vi "Writedata_spectra_normonly.vi"(0 "tdms file in":refnum<k34>, 1 "Aquisition number":i32, 2 "Norm Visible Intensity":cluster{dbl[], dbl[]}(graph)={array[2028 elements], array[2028 elements]}, 3 "tdms error in":errorcluster, 4 "Params":T1) -> (5 "tdms file out":refnum<k34>, 6 "tdms error out":errorcluster)   [LabVIEW 2018]
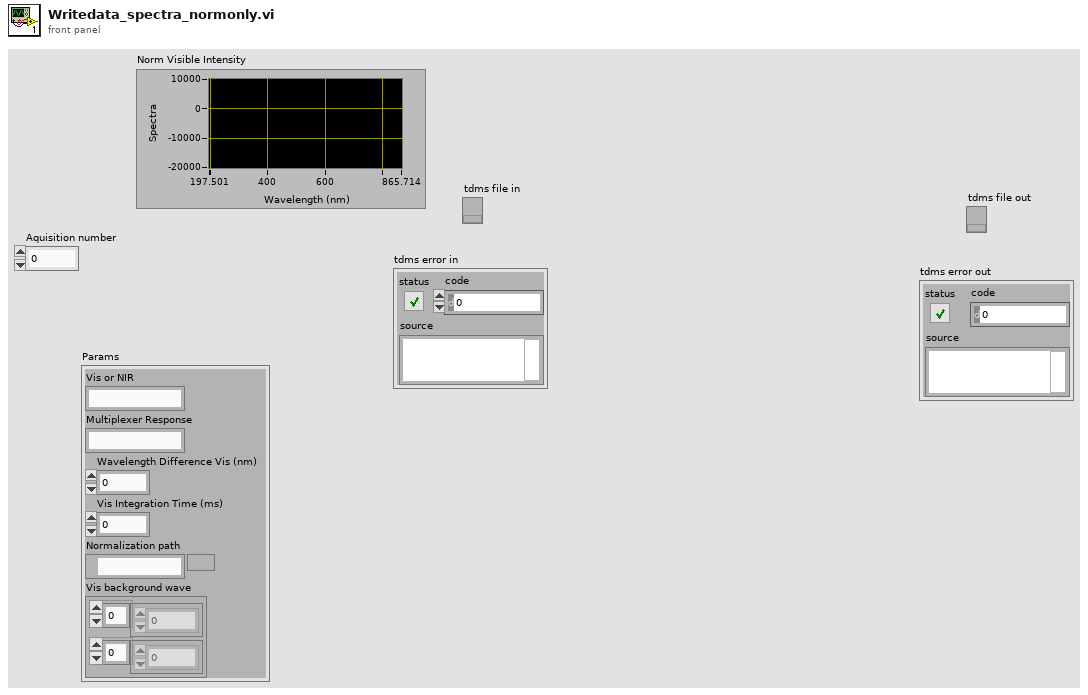
[diagram p1: front panel]
types:
  T1 = cluster{"Vis or NIR":string, "Multiplexer Response":string, "Wavelength Difference Vis (nm)":dbl, "Vis Integration Time (ms)":u32, "Normalization path":path, "Vis background wave":cluster{dbl[], dbl[]}}
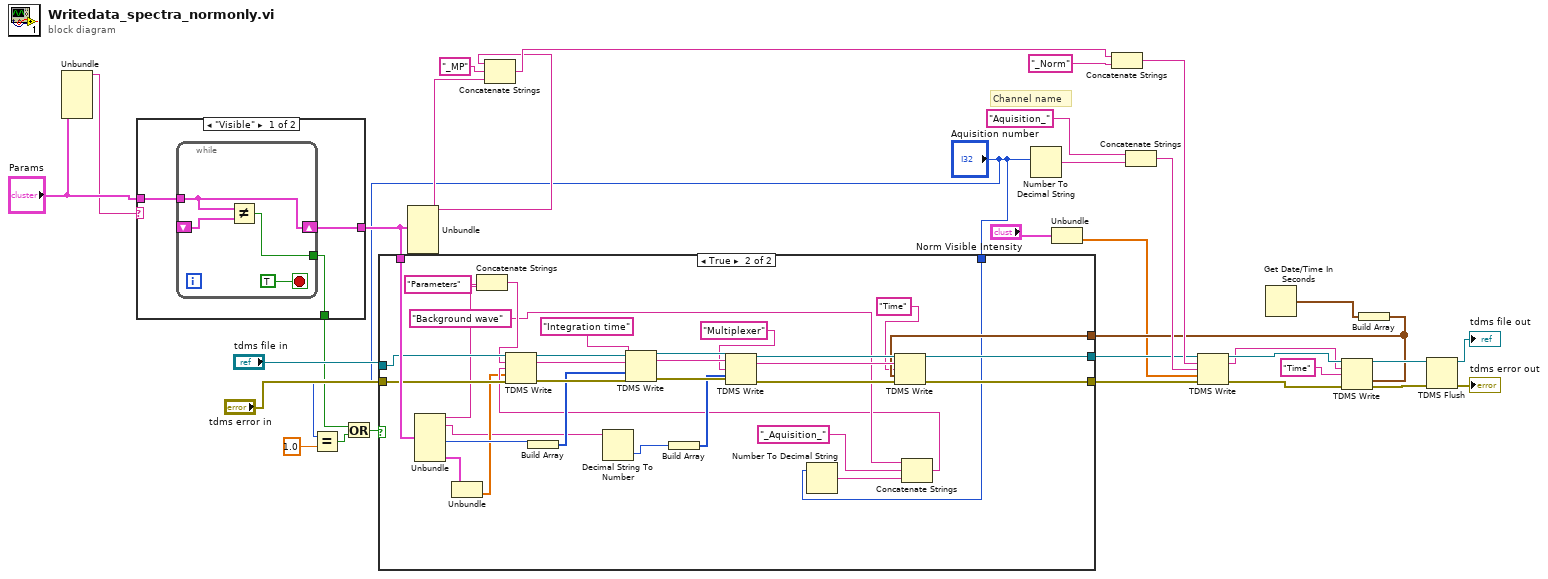
[diagram p0: block diagram]
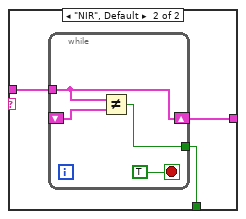
[diagram p2: hidden frame]
diagram:
  # "Channel name"
  n1 = Unbundle("Params") -> ("Vis or NIR"=w6:string)  [unwired: 5 out]
  n2 = case shown="\"Visible\"" w6 {
    tunnel: [w36 w43] -> w1
    tunnel: [w35 w42] -> w11
    tunnel: "Params" -> [w34 w41]
    frame "Visible" {
      n3 = while {
        shift-right: [w39] -> w35
        shift-left: _ -> [w40]
        tunnel: [w38] -> w36
        tunnel: w34 -> [w39]
        stop <- TRUE stop-if-true
        n4 = Not Equal?(x=w39, y=w40) -> (x != y?=w38:bool)
      }
    }
    frame "NIR", Default {
      n5 = while {
        shift-right: [w46] -> w42
        shift-left: _ -> [w47]
        tunnel: [w45] -> w43
        tunnel: w41 -> [w46]
        stop <- TRUE stop-if-true
        n6 = Not Equal?(x=w46, y=w47) -> (x != y?=w45:bool)
      }
    }
  }
  n7 = Equal?(x="Aquisition number", y=1.0) -> (x = y?=w4:bool)
  n8 = Or(x=w1, y=w4) -> (x .or. y?=w5:bool)
  n9 = Unbundle(w11) -> ("Vis or NIR"=w25:string, "Multiplexer Response"=w24:string)  [unwired: 4 out]
  n10 = Concatenate Strings(w25, "_MP" ("group name in (Untitled)"), w24) -> (w29:string)
  n11 = Number To Decimal String(number="Aquisition number") -> (decimal integer string=w30:string)  [unwired: 1 in]
  n12 = Unbundle("Norm Visible Intensity") -> (w8:dbl[])  [unwired: 1 out]
  n13 = Concatenate Strings(w29, "_Norm" ("string")) -> (w23:string)
  n14 = Concatenate Strings("Aquisition_" ("string"), w30) -> (w16:string)
  n15 = Get Date/Time In Seconds() -> (seconds since 1Jan1904=w20:timestamp)
  n16 = Build Array(w20) -> (w10:timestamp[])
  n17 = case shown="True" w5 {
    tunnel: [w49 w64] -> w13
    tunnel: [w48 w63] -> w12
    tunnel: "tdms file in" -> [w49 w81]
    tunnel: "tdms error in" -> [w48 w80]
    tunnel: w11 -> [_ w82]
    tunnel: w10 -> [_ w62]
    tunnel: "Aquisition number" -> [_ w53]
    frame False {
    }
    frame True {
      n18 = Unbundle(w82) -> ("Vis or NIR"=w68:string, "Multiplexer Response"=w51:string, "Vis Integration Time (ms)"=w73:u32, "Vis background wave"=w79:cluster{dbl[], dbl[]})  [unwired: 2 out]
      n19 = Unbundle(w79) -> (w52:dbl[])  [unwired: 1 out]
      n20 = Concatenate Strings("Parameters" ("group name in (Untitled)"), w68) -> (w59:string)
      n21 = Build Array(w73) -> (w72:u32[])
      n22 = Decimal String To Number(string=w51) -> (number=w50:i32)  [unwired: 2 in, 1 out]
      n23 = Build Array(w50) -> (w71:i32[])
      n24 = Number To Decimal String(number=w53) -> (decimal integer string=w57:string)  [unwired: 1 in]
      n25 = Concatenate Strings("Background wave" ("group name in (Untitled)"), "_Aquisition_" ("string"), w57) -> (w54:string)
      n26 = TDMS Write(0:w81, 5:w59, 7:w54, 9:w52, 11:w80) -> (4:w78:refnum<k34>, 6:w70:string, 15:w77:errorcluster)  [unwired: 1 in, 1 out]
      n27 = TDMS Write(0:w78, 5:w70, 7:"Integration time" ("group name in (Untitled)"), 9:w72, 11:w77) -> (4:w76:refnum<k34>, 6:w75:string, 15:w74:errorcluster)  [unwired: 1 in, 1 out]
      n28 = TDMS Write(0:w76, 5:w75, 7:"Multiplexer" ("group name in (Untitled)"), 9:w71, 11:w74) -> (4:w67:refnum<k34>, 6:w66:string, 15:w65:errorcluster)  [unwired: 1 in, 1 out]
      n29 = TDMS Write(0:w67, 5:w66, 7:"Time" ("group name in (Untitled)"), 9:w62, 11:w65) -> (4:w64:refnum<k34>, 15:w63:errorcluster)  [unwired: 1 in, 2 out]
    }
  }
  n30 = TDMS Write(0:w13, 5:w23, 7:w16, 9:w8, 11:w12) -> (4:w22:refnum<k34>, 6:w9:string, 15:w21:errorcluster)  [unwired: 1 in, 1 out]
  n31 = TDMS Write(0:w22, 5:w9, 7:"Time" ("property names"), 9:w10, 11:w21) -> (4:w26:refnum<k34>, 15:w18:errorcluster)  [unwired: 1 in, 2 out]
  n32 = TDMS Flush(4:w18, 7:w26) -> (0:→"tdms error out":errorcluster, 3:→"tdms file out":refnum<k34>)
